vi "ADC Config Panel.vi"(8 "error in":errorcluster, 11 "adc session in":T2={"niScope"={"channel cfg"=[], "sessions"=[], "multi cards"=FALSE, "channels"=0, "type"=enum."n/a", "memory [B/chn]"=0, "ext. clock [Hz]"=0.0, "samples count"=0, "use streaming"=FALSE, "proc setup"={"packet size [smpl]"=0, "current timeout [s]"=0.0, "blk2blk timeout [s]"=0.0, "event time"=timestamp(0 s since 1904-01-01), "temp sampl T [s]"=0.0, "data queue"=refnum, "stop notifier"=refnum, "proc ref"=refnum}, "sample width [B]"=0, "ranges [V]"=[], "trigger setup"={"coupling"=1, "level [V]"=0.0, "slope"=0, "mode"=enum."Immediate"}, "fs [Hz]"=0.0, "bitres [bit]"=0}, "3458A"={"channels"=[], "sync unit"={"VISA"="", "type"=enum."Picotest U6200A"}, "awg unit"={"type"=enum."Agilent 331xxA to 332xxA", "VISA"="", "enable 10MHz ref"=FALSE}, "sync mode"=enum."MASTER-SLAVE, MASTER clocked by TIMER", "streaming mode"=FALSE, "idn mode"=enum."Auto", "sampling mode"=enum."DCV", "Ts [s]"=0.0, "sample memory [B]"=0, "proc setup"={"channel id"=0, "packet size [smpl]"=0, "current timeout [s]"=0.0, "blk2blk timeout [s]"=0.0, "event time"=timestamp(0 s since 1904-01-01), "stop notifier"=refnum, "data queues"=[], "proc refs"=[], "bus semaphore"=refnum}, "sample size [B]"=0, "sample count"=0, "aux data"={"channel id"=0, "valid?"=[], "gain [V]"=[], "timestamp [s]"=[], "Ts [s]"=0.0, "abs timestamp"=timestamp(0 s since 1904-01-01), "t [deg C]"=[]}, "ranges [V]"=[], "aperture [s]"=0.0, "LEVEL trigger"={"edge"=enum."POS", "level [V]"=0.0, "coupling"=enum."DC"}, "trigger mode"=enum."AUTO", "measure temp.?"=FALSE, "disp mesages"=[], "shared bus?"=FALSE, "disable display?"=FALSE, "aper mode"=enum."Manual", "aper rules"=[]}, "dsdll"={"dsdll"={"dsdll path"=path "", "dsdll handle"=[], "output devices"=[], "capture devices"=[]}, "channels"=0, "device id"=0, "channel idns"=[], "proc setup"={"packet size [smpl]"=0, "current timeout [s]"=0.0, "blk2blk timeout [s]"=0.0, "event time"=timestamp(0 s since 1904-01-01), "data queue"=refnum, "stop notifier"=refnum, "proc ref"=refnum}, "samples count"=0, "fs [Hz]"=0.0}, "type"=enum."niScope", "channel idn str"=[], "aux instr idn str"=[], "modified?"=FALSE, "simadc"={"channels"=[], "range [V]"=0.0, "Ts step [s]"=0.0, "time [s]"=0.0, "fs [Hz]"=0.0, "count"=0, "smpl offset"=0, "set count"=0, "bit res"=0}, "force rst?"=FALSE, "exit mode"=enum."Immediate reset", "exit dly"=0.0, "exit tmr"=timestamp(0 s since 1904-01-01), "busy?"=FALSE, "accessed?"=FALSE, "QuADC session"={"channel cfg"=[], "sessions"=[], "multi cards"=FALSE, "channels"=0, "type"=enum."n/a", "memory [B/chn]"=0, "ext. clock [Hz]"=0.0, "samples count"=0, "use streaming"=FALSE, "proc setup"={"packet size [smpl]"=0, "current timeout [s]"=0.0, "blk2blk timeout [s]"=0.0, "event time"=timestamp(0 s since 1904-01-01), "temp sampl T [s]"=0.0, "data queue"=refnum, "stop notifier"=refnum, "proc ref"=refnum}, "sample width [B]"=0, "ranges [V]"=[], "trigger setup"={"coupling"=1, "level [V]"=0.0, "slope"=0, "mode"=enum."Immediate"}, "fs [Hz]"=0.0, "bitres [bit]"=0}} {"QuADC session"."trigger setup"."level [V]" format="%.2f"; "QuADC session"."trigger setup"."coupling" items=["AC"=0, "DC"=1, "HF Reject"=3, "LF Reject"=4, "AC Plus HF Reject"=1001]; "QuADC session"."channel cfg"."Clock fr. (Hz)" min=0.0 format="%#_9p"; "QuADC session"."channel cfg"."Number of JJ" min=1; "QuADC session"."channel cfg"."Range [Vpk]" min=0.0; "QuADC session"."channel cfg"."Channel" min=0; "3458A"."channels"."Range [Vpk]" min=0.0; "niScope"."trigger setup"."level [V]" format="%.2f"; "niScope"."trigger setup"."coupling" items=["AC"=0, "DC"=1, "HF Reject"=3, "LF Reject"=4, "AC Plus HF Reject"=1001]; "niScope"."channel cfg"."Range [Vpk]" min=0.0; "niScope"."channel cfg"."Channel" min=0}) -> (0 "error out":errorcluster, 3 "adc session out":T2={"niScope"={"channel cfg"=[], "sessions"=[], "multi cards"=FALSE, "channels"=0, "type"=enum."n/a", "memory [B/chn]"=0, "ext. clock [Hz]"=0.0, "samples count"=0, "use streaming"=FALSE, "proc setup"={"packet size [smpl]"=0, "current timeout [s]"=0.0, "blk2blk timeout [s]"=0.0, "event time"=timestamp(0 s since 1904-01-01), "temp sampl T [s]"=0.0, "data queue"=refnum, "stop notifier"=refnum, "proc ref"=refnum}, "sample width [B]"=0, "ranges [V]"=[], "trigger setup"={"coupling"=1, "level [V]"=0.0, "slope"=0, "mode"=enum."Immediate"}, "fs [Hz]"=0.0, "bitres [bit]"=0}, "3458A"={"channels"=[], "sync unit"={"VISA"="", "type"=enum."Picotest U6200A"}, "awg unit"={"type"=enum."Agilent 331xxA to 332xxA", "VISA"="", "enable 10MHz ref"=FALSE}, "sync mode"=enum."MASTER-SLAVE, MASTER clocked by TIMER", "streaming mode"=FALSE, "idn mode"=enum."Auto", "sampling mode"=enum."DCV", "Ts [s]"=0.0, "sample memory [B]"=0, "proc setup"={"channel id"=0, "packet size [smpl]"=0, "current timeout [s]"=0.0, "blk2blk timeout [s]"=0.0, "event time"=timestamp(0 s since 1904-01-01), "stop notifier"=refnum, "data queues"=[], "proc refs"=[], "bus semaphore"=refnum}, "sample size [B]"=0, "sample count"=0, "aux data"={"channel id"=0, "valid?"=[], "gain [V]"=[], "timestamp [s]"=[], "Ts [s]"=0.0, "abs timestamp"=timestamp(0 s since 1904-01-01), "t [deg C]"=[]}, "ranges [V]"=[], "aperture [s]"=0.0, "LEVEL trigger"={"edge"=enum."POS", "level [V]"=0.0, "coupling"=enum."DC"}, "trigger mode"=enum."AUTO", "measure temp.?"=FALSE, "disp mesages"=[], "shared bus?"=FALSE, "disable display?"=FALSE, "aper mode"=enum."Manual", "aper rules"=[]}, "dsdll"={"dsdll"={"dsdll path"=path "", "dsdll handle"=[], "output devices"=[], "capture devices"=[]}, "channels"=0, "device id"=0, "channel idns"=[], "proc setup"={"packet size [smpl]"=0, "current timeout [s]"=0.0, "blk2blk timeout [s]"=0.0, "event time"=timestamp(0 s since 1904-01-01), "data queue"=refnum, "stop notifier"=refnum, "proc ref"=refnum}, "samples count"=0, "fs [Hz]"=0.0}, "type"=enum."niScope", "channel idn str"=[], "aux instr idn str"=[], "modified?"=FALSE, "simadc"={"channels"=[], "range [V]"=0.0, "Ts step [s]"=0.0, "time [s]"=0.0, "fs [Hz]"=0.0, "count"=0, "smpl offset"=0, "set count"=0, "bit res"=0}, "force rst?"=FALSE, "exit mode"=enum."Immediate reset", "exit dly"=0.0, "exit tmr"=timestamp(0 s since 1904-01-01), "busy?"=FALSE, "accessed?"=FALSE, "QuADC session"={"channel cfg"=[], "sessions"=[], "multi cards"=FALSE, "channels"=0, "type"=enum."n/a", "memory [B/chn]"=0, "ext. clock [Hz]"=0.0, "samples count"=0, "use streaming"=FALSE, "proc setup"={"packet size [smpl]"=0, "current timeout [s]"=0.0, "blk2blk timeout [s]"=0.0, "event time"=timestamp(0 s since 1904-01-01), "temp sampl T [s]"=0.0, "data queue"=refnum, "stop notifier"=refnum, "proc ref"=refnum}, "sample width [B]"=0, "ranges [V]"=[], "trigger setup"={"coupling"=1, "level [V]"=0.0, "slope"=0, "mode"=enum."Immediate"}, "fs [Hz]"=0.0, "bitres [bit]"=0}} {"QuADC session"."trigger setup"."level [V]" format="%.2f"; "QuADC session"."trigger setup"."coupling" items=["AC"=0, "DC"=1, "HF Reject"=3, "LF Reject"=4, "AC Plus HF Reject"=1001]; "QuADC session"."channel cfg"."Clock fr. (Hz)" min=0.0 format="%#_9p"; "QuADC session"."channel cfg"."Number of JJ" min=1; "QuADC session"."channel cfg"."Range [Vpk]" min=0.0; "QuADC session"."channel cfg"."Channel" min=0; "3458A"."channels"."Range [Vpk]" min=0.0; "niScope"."trigger setup"."level [V]" format="%.2f"; "niScope"."trigger setup"."coupling" items=["AC"=0, "DC"=1, "HF Reject"=3, "LF Reject"=4, "AC Plus HF Reject"=1001]; "niScope"."channel cfg"."Range [Vpk]" min=0.0; "niScope"."channel cfg"."Channel" min=0})   [LabVIEW 2018]
doc: "Configuration panel for digitizer."
uses:
  drivers/niScope/niScope Virtual Channel Config.ctl
  drivers/niScope/niScope Virtual Channel Mode.ctl
  drivers/niScope/niScope Virtual Channel Input Z.ctl
  drivers/niScope/niScope Virtual Channel Coupling.ctl
  ADC Type.ctl
  drivers/DMM/3458A Virtual Channel Config.ctl
  drivers/AWG/AWG Type.ctl
  drivers/DMM/3458A Idn Mode.ctl
  drivers/Counter/Counter Type.ctl
  drivers/DMM/3458A Digitizing Low Levels/Configure/Sampling Mode.ctl
  drivers/DMM/3458A Sync Mode.ctl
  ADC Session.ctl
  drivers/niScope/niScope Session.ctl
  drivers/niScope/niScope Type.ctl
  drivers/niScope/niScope Digitizing Process Options.ctl
  drivers/niScope/niScope Data Packet.ctl
  drivers/niScope/niScope Trigger Setup.ctl
  <instrlib>/niScope/Controls/niScope trigger coupling.ctl
  <instrlib>/niScope/Controls/niScope trigger slope.ctl
  drivers/DMM/3458A Digitizer Session.ctl
  drivers/Counter/Counter Session.ctl
  drivers/AWG/AWG Session.ctl
  drivers/DMM/3458A Digitizing Process Options.ctl
  drivers/DMM/3458A Data Packet.ctl
  drivers/DMM/3458A Aux Record Data.ctl
  drivers/DMM/3458A Digitizing Low Levels/Configure/Level Setup.ctl
  drivers/DMM/3458A Digitizing Low Levels/Configure/First Sample Trigger.ctl
  drivers/DMM/3458A Aperture Selection Mode.ctl
  drivers/dsdll/DSDLL Session.ctl
  drivers/dsdll/dsdll source distribution/dsdll_instance.ctl
  drivers/dsdll/dsdll source distribution/dsdll_device_record.ctl
  drivers/dsdll/DSDLL Process Config.ctl
  drivers/dsdll/DSDLL Data Packet.ctl
  drivers/simulated_adc/SimAdc Config.ctl
  drivers/simulated_adc/SimAdc Channel Cfg.ctl
  ADC On Close Action.ctl
  drivers/Quatsch_driver/QuADCDriver/QuADC Session.ctl
  drivers/Quatsch_driver/QuADCDriver/QuADC Virtual Channel Config.ctl
  drivers/Quatsch_driver/QuADCDriver/QuADC Virtual Channel Mode.ctl
  drivers/Quatsch_driver/QuADCDriver/QuADC Virtual Channel Input Z.ctl
  drivers/Quatsch_driver/QuADCDriver/QuADC Virtual Channel Coupling.ctl
  drivers/Quatsch_driver/QuADCDriver/QuADC Type.ctl
  drivers/Quatsch_driver/QuADCDriver/QuADC Digitizing Process Options.ctl
  drivers/Quatsch_driver/QuADCDriver/QuADC Data Packet.ctl
  drivers/Quatsch_driver/QuADCDriver/QuADC Trigger Setup.ctl
  varilib/SGUI Assign References Mode.ctl
  varilib/SGUI Assign Multiple Strings With Tags By Label.vi
  drivers/DMM/3458A Virtual Digitizer.lvlib
  drivers/Counter/Counter.lvlib
  drivers/AWG/AWG.lvlib
  drivers/DMM/3458A Digitizing Low Levels/3458A Digitizing Low Levels.lvlib
  varilib/varilib.lvlib
  drivers/niScope/niScope Virtual Digitizer.lvlib
  drivers/dsdll/DSDLL Virtual Digitizer.lvlib
  drivers/Quatsch_driver/QuADCDriver/QuADC Virtual Digitizer.lvlib
  drivers/dsdll/dsdll source distribution/dsdll.lvlib
panel:
  in  "tc on exit":enum32{"Page 1"}(tab)
  in  "exit delay":dbl=30.0 caption="Delay [s]"
  in  "exit mode":T1 caption="On device close"
  in  "force rst":bool caption="Force reset on open"
  in  "btn selfcal":bool
  in  "tc idn":enum32{"Page 1"}(tab)
  out "adcstr":string caption="Identification/Status:"
  in  "btn test":bool
  in  "btn cancel":bool
  in  "btn ok":bool
  in  "tc type":enum32{"Page 1"}(tab)
  out "Description":string
  in  "Digitizer type":T32
  in  "tc cfg":T43(tab)
  in  "btn rem last niScope":bool
  in  "niSc streaming":bool caption="Use streaming mode"
  in  "niSc ext clock":dbl caption="External clock [Hz]" format="%#_6p"
  in  "btn clr niScope":bool
  in  "niSc channels":T4[](array[typedef]) caption="ADC Channels" {"Range [Vpk]" min=0.0; "Channel" min=0}
  in  "dmm aper mode":T27 caption="Aperture selection mode"
  in  "dmm aper rules":string[][](table) caption="Aperture auto selection rules"
  in  "dmm disable disp":bool caption="Disable display"
  in  "btn rem last dmm":bool
  in  "dmm meas t":bool caption="Measure temperature"
  in  "dmm stream":bool caption="Use streaming mode"
  in  "dmm sync mode":T19 caption="Synchronization mode"
  in  "counter VISA":refnum<visa-resource-name> caption="Counter VISA"
  in  "AWG VISA":refnum<visa-resource-name>
  in  "counter type":T16 caption="Counter type"
  in  "AWG ext ref":bool caption="Use external 10 MHz for AWG"
  in  "AWG type":T18
  in  "DMM Channels":T14[](array[typedef]) {"Range [Vpk]" min=0.0}
  in  "btn clr dmm":bool
  in  "dmm idn mode":T20 caption="DMM descriptor mode"
  in  "dmm smpl mode":T21 caption="DMM digitizing mode"
  in  "btn dsdll enum":bool
  in  "dsdll channels":i32=1 caption="Channels count (1 or 2)" min=1 max=2 step=1
  in  "dsdll capt devs":u16(ring) caption="Capture devices"
  in  "simadc bitres":i32=16 caption="ADC resolution [bit]"
  in  "Range [V]":dbl
  in  "Sampling period step [s]":dbl
  in  "btn sim clr":bool caption="Clear List"
  in  "simadc chn cfg":T34[](array[typedef]) caption="Channel signal definitions"
  in  "QuADC channels":T36[](array[typedef])=[{"Channel"=0, "Mode"=enum."Single ended", "Input Z"=enum."1 MOhm", "Coupling"=enum."DC", "Range [Vpk]"=1.0, "btn clr"=FALSE, "btn up"=FALSE, "btn down"=FALSE, "IP address A"=127, "IP address B"=0, "IP address C"=0, "IP address D"=1, "Port"=8888, "Number of JJ"=1000, "Clock fr. (Hz)"=5000000000.0}] {"Clock fr. (Hz)" min=0.0 format="%#_9p"; "Number of JJ" min=1; "Range [Vpk]" min=0.0; "Channel" min=0}
  # "IP Address"
  # "."
  # "."
  # "."
  # ":"
  # "IP Address"
  # "."
  # "."
  # "."
  # ":"
  # "- Use 0 for internal clock"
  # "Streaming mode is used always."
  # "IP Address"
  # "."
  # "."
  # "."
  # ":"
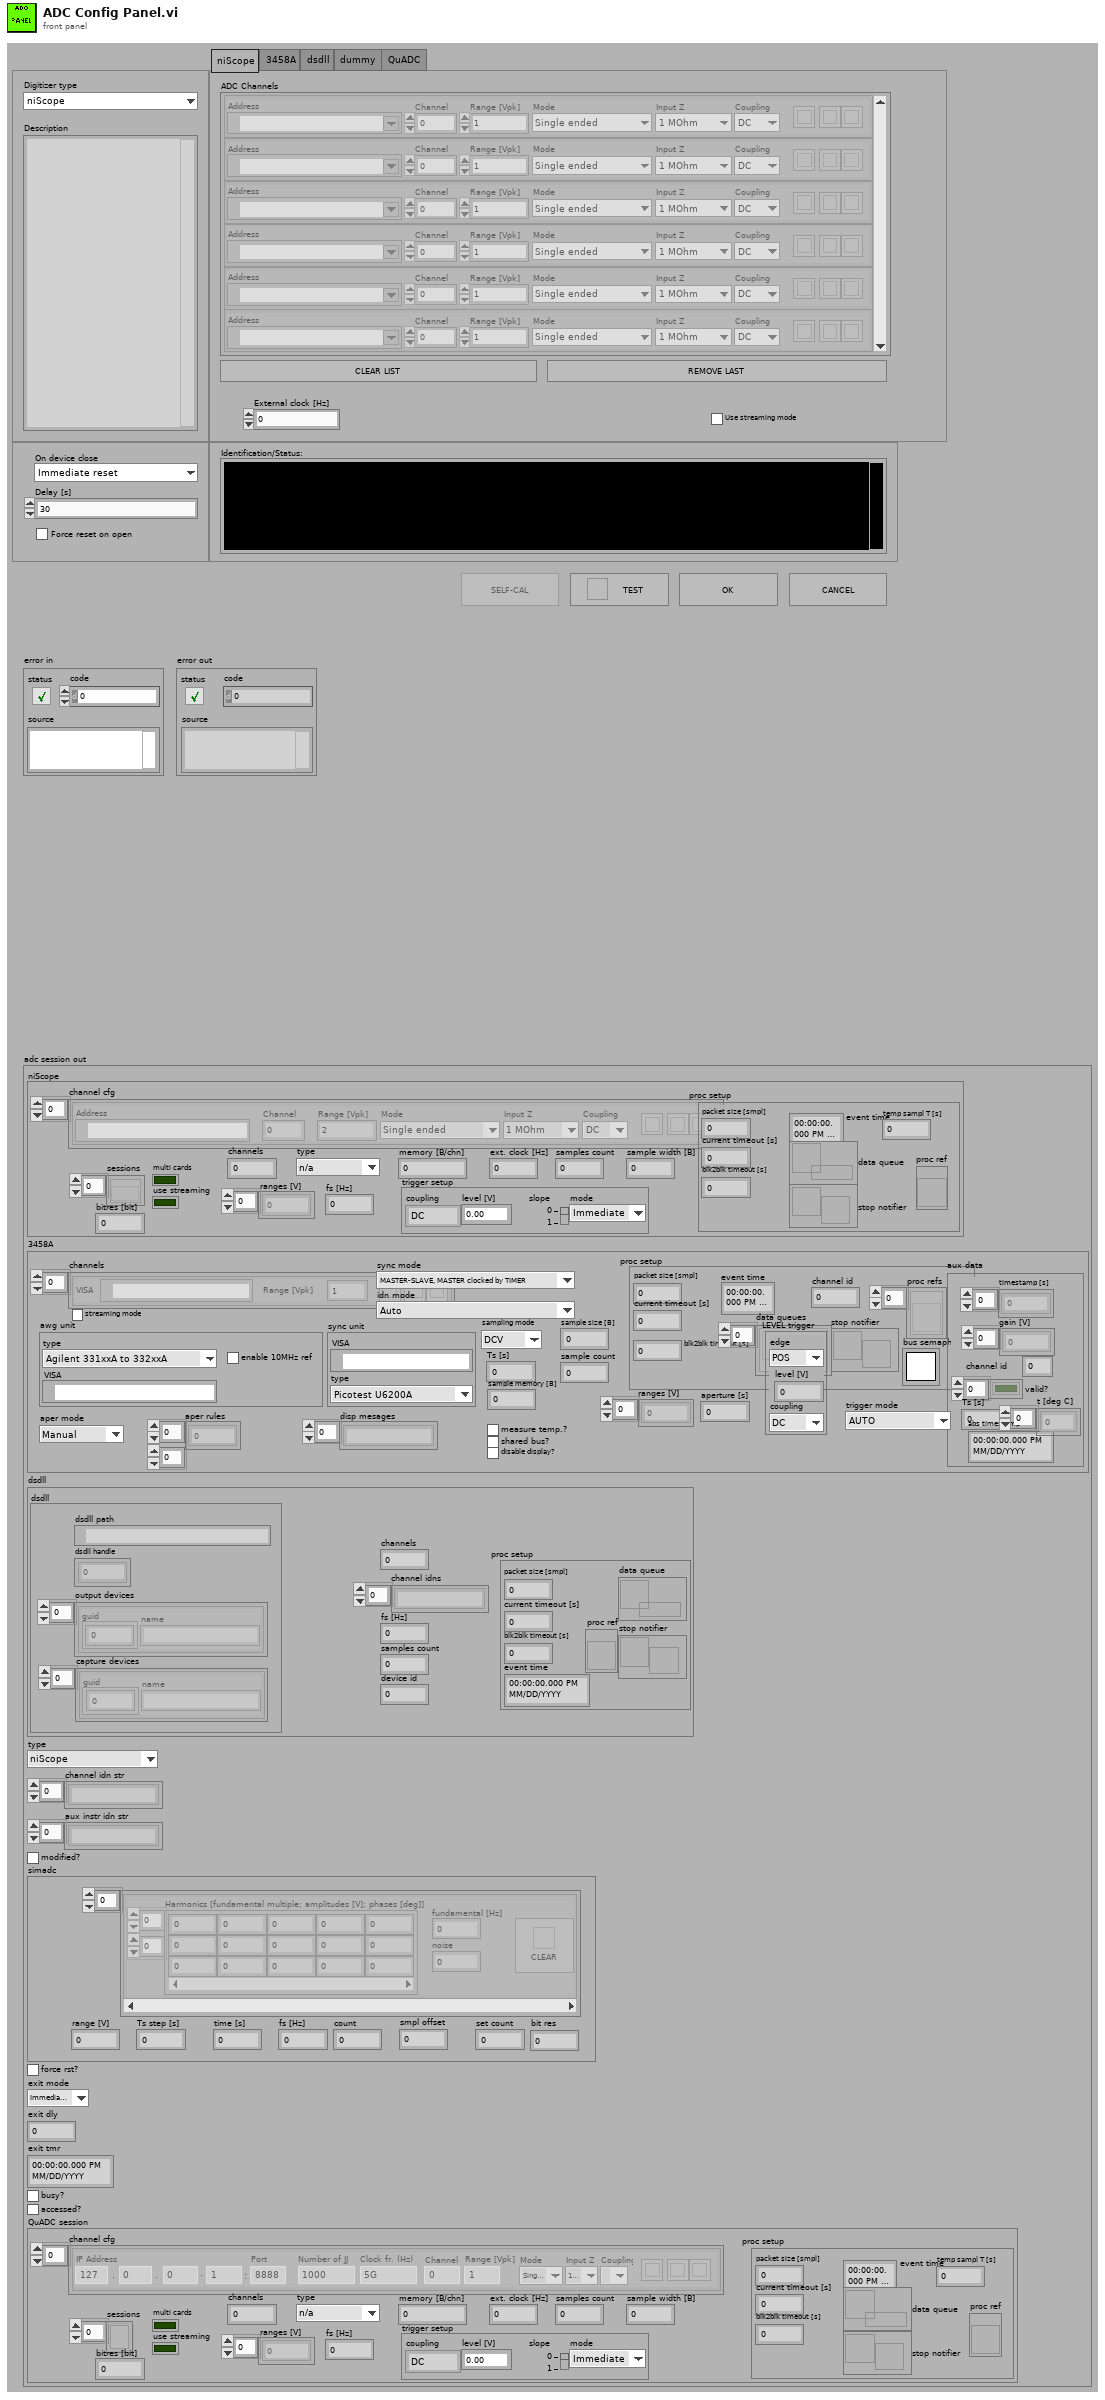
[diagram p1: front panel]
types:
  T1 = typedef "ADC On Close Action.ctl" = enum16{"Immediate reset", "Delayed reset"}
  T2 = typedef "ADC Session.ctl" = cluster{"niScope":T3, "3458A":T13, "dsdll":T28, "type":T32, "channel idn str":string[], "aux instr idn str":string[], "modified?":bool, "simadc":T33, "force rst?":bool, "exit mode":T1, "exit dly":dbl, "exit tmr":timestamp, "busy?":bool, "accessed?":bool, "QuADC session":T35}
  T3 = typedef "niScope Virtual Digitizer.lvlib/niScope Session.ctl" = cluster{"channel cfg":T4[], "sessions":refnum<k20>[], "multi cards":bool, "channels":i32, "type":T8, "memory [B/chn]":i32, "ext. clock [Hz]":dbl, "samples count":i64, "use streaming":bool, "proc setup":T9, "sample width [B]":i32, "ranges [V]":dbl[], "trigger setup":T10, "fs [Hz]":dbl, "bitres [bit]":i32}
  T4 = typedef "niScope Virtual Digitizer.lvlib/niScope Virtual Channel Config.ctl" = cluster{"Address":refnum<k15>, "Channel":i32, "Mode":T5, "Input Z":T6, "Coupling":T7, "Range [Vpk]":dbl, "btn clr":bool, "btn up":bool, "btn down":bool}
  T5 = typedef "niScope Virtual Digitizer.lvlib/niScope Virtual Channel Mode.ctl" = enum16{"Single ended", "Unbal. differential", "Differential"}
  T6 = typedef "niScope Virtual Digitizer.lvlib/niScope Virtual Channel Input Z.ctl" = enum16{"1 MOhm", "50 Ohm"}
  T7 = typedef "niScope Virtual Digitizer.lvlib/niScope Virtual Channel Coupling.ctl" = enum16{"AC", "DC", "GND"}
  T8 = typedef "niScope Virtual Digitizer.lvlib/niScope Type.ctl" = enum16{"n/a", "5922"}
  T9 = typedef "niScope Virtual Digitizer.lvlib/niScope Digitizing Process Options.ctl" = cluster{"packet size [smpl]":i64, "current timeout [s]":dbl, "blk2blk timeout [s]":dbl, "event time":timestamp, "temp sampl T [s]":dbl, "data queue":refnum<queue>, "stop notifier":refnum<notifier>, "proc ref":refnum<vi>}
  T10 = typedef "niScope Virtual Digitizer.lvlib/niScope Trigger Setup.ctl" = cluster{"coupling":T11, "level [V]":dbl, "slope":T12, "mode":enum16{"Immediate", "External", "Level"}}
  T11 = typedef "niScope trigger coupling.ctl" = u16
  T12 = typedef "niScope trigger slope.ctl" = i32
  T13 = typedef "3458A Virtual Digitizer.lvlib/3458A Digitizer Session.ctl" = cluster{"channels":T14[], "sync unit":T15, "awg unit":T17, "sync mode":T19, "streaming mode":bool, "idn mode":T20, "sampling mode":T21, "Ts [s]":dbl, "sample memory [B]":i32, "proc setup":T22, "sample size [B]":i32, "sample count":i32, "aux data":T24, "ranges [V]":dbl[], "aperture [s]":dbl, "LEVEL trigger":T25, "trigger mode":T26, "measure temp.?":bool, "disp mesages":string[], "shared bus?":bool, "disable display?":bool, "aper mode":T27, "aper rules":dbl[][]}
  T14 = typedef "3458A Virtual Digitizer.lvlib/3458A Virtual Channel Config.ctl" = cluster{"VISA":refnum<visa-resource-name>, "Range [Vpk]":dbl, "btn clr":bool, "btn up":bool, "btn down":bool}
  T15 = typedef "Counter.lvlib/Counter Session.ctl" = cluster{"VISA":refnum<visa-resource-name>, "type":T16}
  T16 = typedef "Counter.lvlib/Counter Type.ctl" = enum16{"Picotest U6200A", "dummy"}
  T17 = typedef "AWG.lvlib/AWG Session.ctl" = cluster{"type":T18, "VISA":refnum<visa-resource-name>, "enable 10MHz ref":bool}
  T18 = typedef "AWG.lvlib/AWG Type.ctl" = enum16{"Agilent 331xxA to 332xxA", "Agilent 335xxA to 336xxA", "Tektronix AFG3101C", "dummy"}
  T19 = typedef "3458A Virtual Digitizer.lvlib/3458A Sync Mode.ctl" = enum16{"MASTER-SLAVE, MASTER clocked by TIMER", "MASTER-SLAVE, MASTER clocked by AWG", "ALL clocked by AWG", "MASTER-SLAVE, ALL clocked by TIMER", "ALL clocked by AWG with DFLL"}
  T20 = typedef "3458A Virtual Digitizer.lvlib/3458A Idn Mode.ctl" = enum16{"Auto", "Sequential (chn A, chn B, ...)", "From calibration string"}
  T21 = typedef "3458A Virtual Digitizer.lvlib/3458A Digitizing Low Levels.lvlib/Sampling Mode.ctl" = enum16{"DCV", "DSDC", "DSAC"}
  T22 = typedef "3458A Virtual Digitizer.lvlib/3458A Digitizing Process Options.ctl" = cluster{"channel id":i32, "packet size [smpl]":i32, "current timeout [s]":dbl, "blk2blk timeout [s]":dbl, "event time":timestamp, "stop notifier":refnum<notifier>, "data queues":refnum<queue>[], "proc refs":refnum<vi>[], "bus semaphore":T23}
  T23 = typedef "Semaphore RefNum" = refnum<k1>
  T24 = typedef "3458A Virtual Digitizer.lvlib/3458A Aux Record Data.ctl" = cluster{"channel id":i32, "valid?":bool[], "gain [V]":dbl[], "timestamp [s]":dbl[], "Ts [s]":dbl, "abs timestamp":timestamp, "t [deg C]":dbl[]}
  T25 = typedef "3458A Virtual Digitizer.lvlib/3458A Digitizing Low Levels.lvlib/Level Setup.ctl" = cluster{"edge":enum16{"POS", "NEG"}, "level [V]":dbl, "coupling":enum16{"DC", "AC"}}
  T26 = typedef "3458A Virtual Digitizer.lvlib/3458A Digitizing Low Levels.lvlib/First Sample Trigger.ctl" = enum16{"AUTO", "EXT", "SYN", "SGL", "HOLD", "LEVEL"}
  T27 = typedef "3458A Virtual Digitizer.lvlib/3458A Aperture Selection Mode.ctl" = enum16{"Manual", "Maximum", "Table"}
  T28 = typedef "DSDLL Virtual Digitizer.lvlib/DSDLL Session.ctl" = cluster{"dsdll":T29, "channels":i32, "device id":i32, "channel idns":string[], "proc setup":T31, "samples count":i32, "fs [Hz]":dbl}
  T29 = typedef "dsdll.lvlib/dsdll_instance.ctl" = cluster{"dsdll path":path, "dsdll handle":u8[], "output devices":T30[], "capture devices":T30[]}
  T30 = typedef "dsdll.lvlib/dsdll_device_record.ctl" = cluster{"guid":u8[], "name":string}
  T31 = typedef "DSDLL Virtual Digitizer.lvlib/DSDLL Process Config.ctl" = cluster{"packet size [smpl]":i32, "current timeout [s]":dbl, "blk2blk timeout [s]":dbl, "event time":timestamp, "data queue":refnum<queue>, "stop notifier":refnum<notifier>, "proc ref":refnum<vi>}
  T32 = typedef "ADC Type.ctl" = enum16{"niScope", "3458A", "DirectSound DLL", "dummy", "QuADC"}
  T33 = typedef "SimAdc Config.ctl" = cluster{"channels":T34[], "range [V]":dbl, "Ts step [s]":dbl, "time [s]":dbl, "fs [Hz]":dbl, "count":i64, "smpl offset":i64, "set count":i64, "bit res":i32}
  T34 = typedef "SimAdc Channel Cfg.ctl" = cluster{"harmonics":dbl[][], "btn clear":bool, "noise":dbl, "fundamental [Hz]":dbl}
  T35 = typedef "QuADC Virtual Digitizer.lvlib/QuADC Session.ctl" = cluster{"channel cfg":T36[], "sessions":refnum<k5>[], "multi cards":bool, "channels":i32, "type":T40, "memory [B/chn]":i32, "ext. clock [Hz]":dbl, "samples count":i64, "use streaming":bool, "proc setup":T41, "sample width [B]":i32, "ranges [V]":dbl[], "trigger setup":T42, "fs [Hz]":dbl, "bitres [bit]":i32}
  T36 = typedef "QuADC Virtual Digitizer.lvlib/QuADC Virtual Channel Config.ctl" = cluster{"Channel":i32, "Mode":T37, "Input Z":T38, "Coupling":T39, "Range [Vpk]":dbl, "btn clr":bool, "btn up":bool, "btn down":bool, "IP address A":u8, "IP address B":u8, "IP address C":u8, "IP address D":u8, "Port":u16, "Number of JJ":u32, "Clock fr. (Hz)":dbl}
  T37 = typedef "QuADC Virtual Digitizer.lvlib/QuADC Virtual Channel Mode.ctl" = enum16{"Single ended", "Unbal. differential", "Differential"}
  T38 = typedef "QuADC Virtual Digitizer.lvlib/QuADC Virtual Channel Input Z.ctl" = enum16{"1 MOhm", "50 Ohm"}
  T39 = typedef "QuADC Virtual Digitizer.lvlib/QuADC Virtual Channel Coupling.ctl" = enum16{"AC", "DC", "GND"}
  T40 = typedef "QuADC Virtual Digitizer.lvlib/QuADC Type.ctl" = enum16{"n/a", "v1"}
  T41 = typedef "QuADC Virtual Digitizer.lvlib/QuADC Digitizing Process Options.ctl" = cluster{"packet size [smpl]":i64, "current timeout [s]":dbl, "blk2blk timeout [s]":dbl, "event time":timestamp, "temp sampl T [s]":dbl, "data queue":refnum<queue>, "stop notifier":refnum<notifier>, "proc ref":refnum<vi>}
  T42 = typedef "QuADC Virtual Digitizer.lvlib/QuADC Trigger Setup.ctl" = cluster{"coupling":T11, "level [V]":dbl, "slope":T12, "mode":enum16{"Immediate", "External", "Level"}}
  T43 = enum32{"niScope", "3458A", "dsdll", "dummy", "QuADC"}
  T44 = typedef "varilib.lvlib/SGUI Assign References Mode.ctl" = enum16{"Add to stack", "Overwrite", "Release last", "Release ID"}
  T45 = typedef "ADC Capabilities.ctl" = cluster{"max samples count":i64, "max fs [Hz]":ext, "min fs [Hz]":ext, "Ts step [s]":ext, "max Ts [s]":ext, "min Ts [s]":ext, "allows streaming?":bool, "streaming on?":bool, "has level trig?":bool, "has ext trig?":bool, "has aperture?":bool, "aper min [s]":dbl, "aper max [s]":dbl, "channels count":i32, "has ranges?":bool, "has temperature?":bool, "has temperature log?":bool, "has selfcal?":bool, "fs step [Hz]":ext, "smpl rate step mode":T46}
  T46 = typedef "ADC Sampling Rate Step Mode.ctl" = enum16{"const period", "const frequency"}
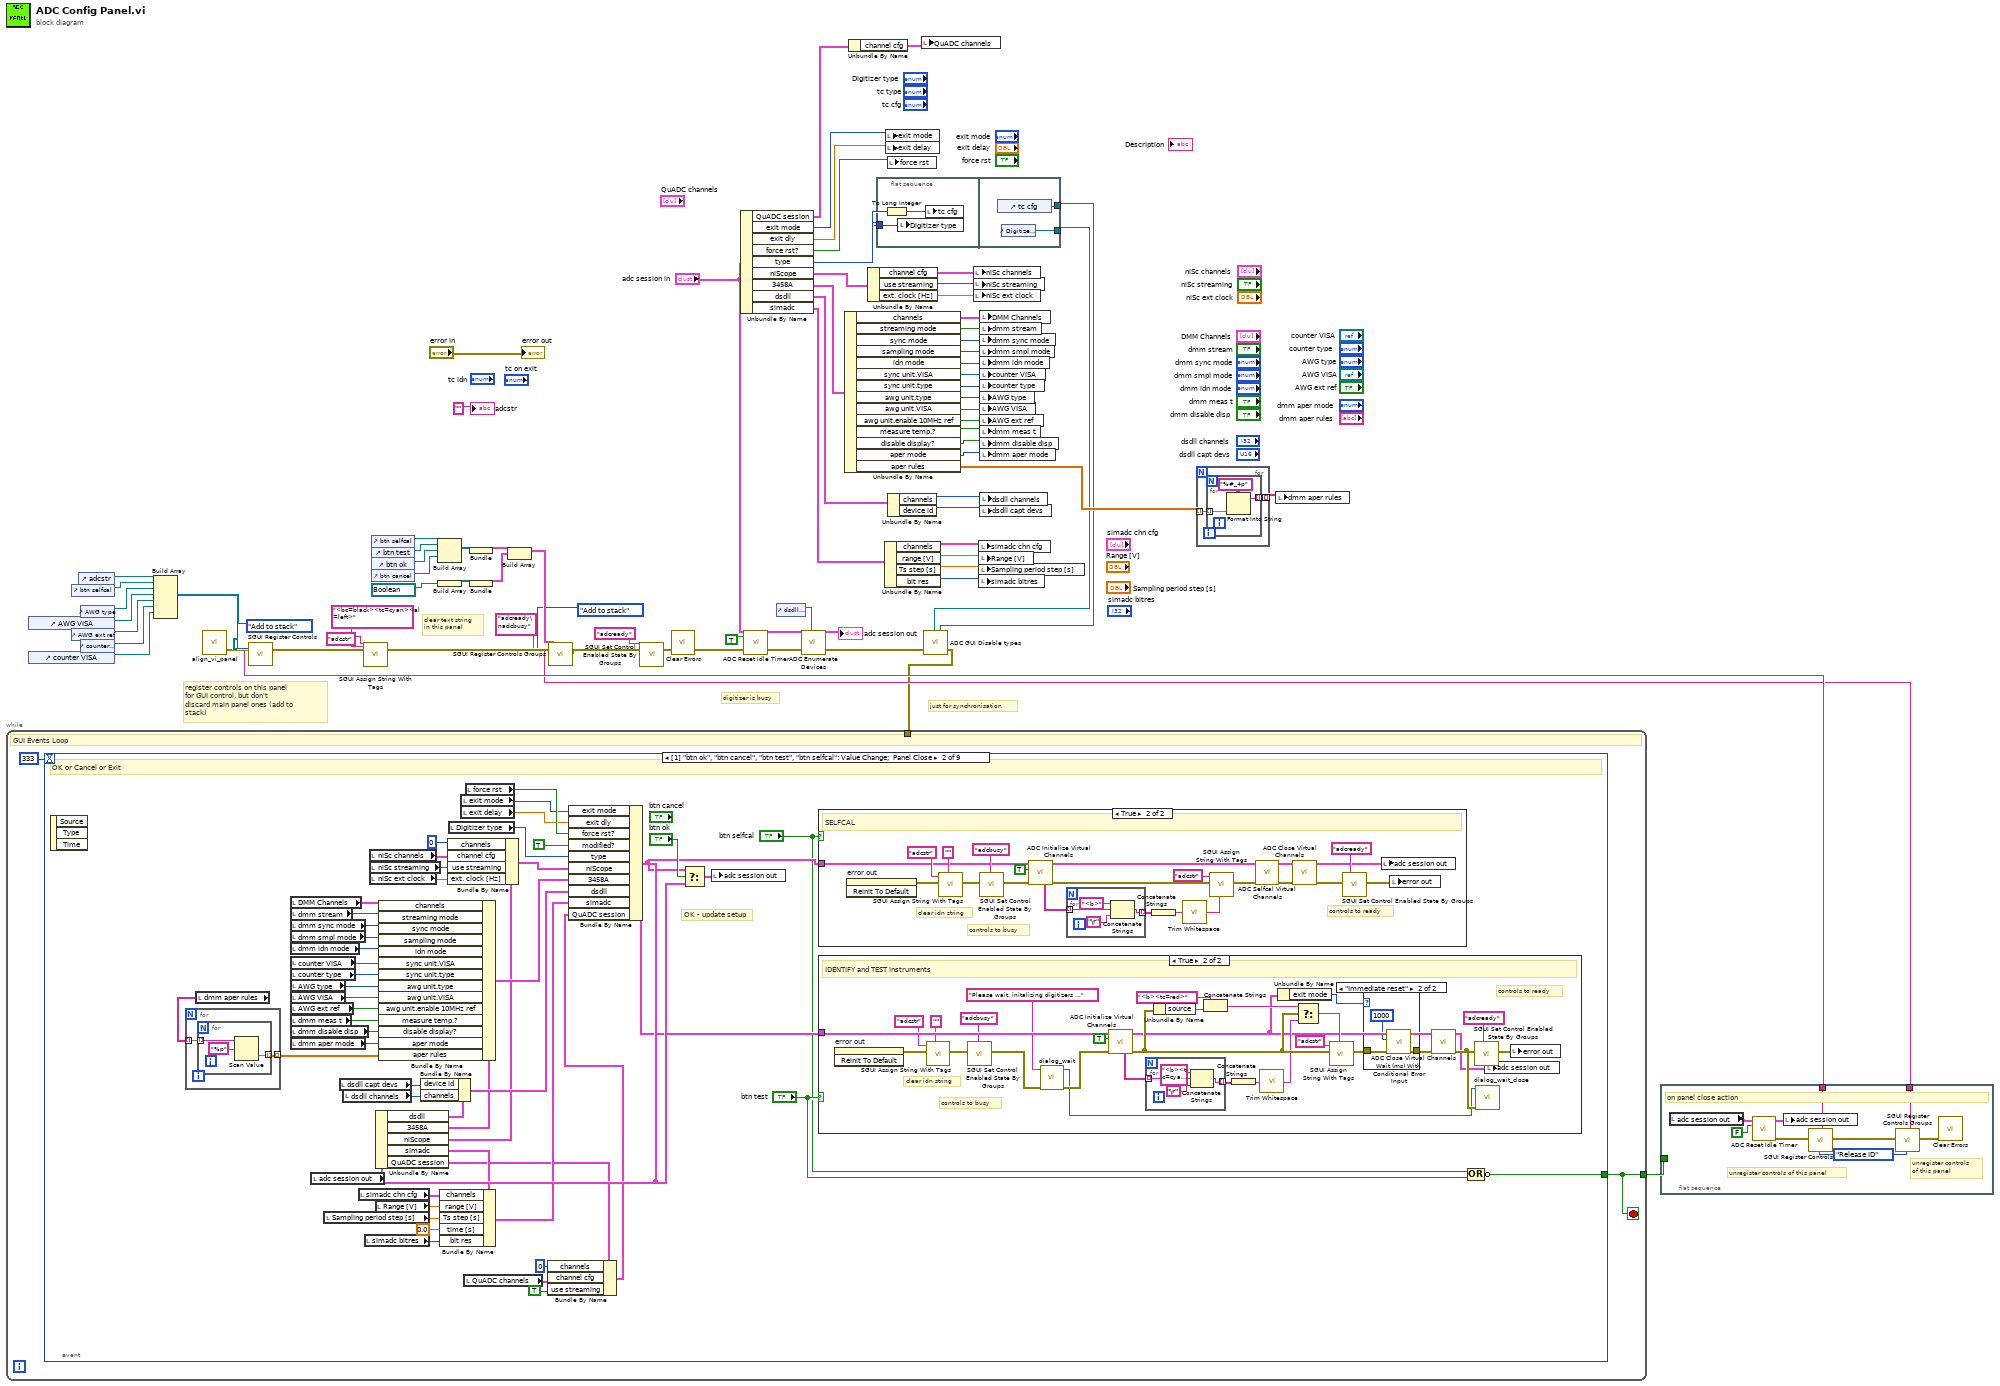
[diagram p0: block diagram]
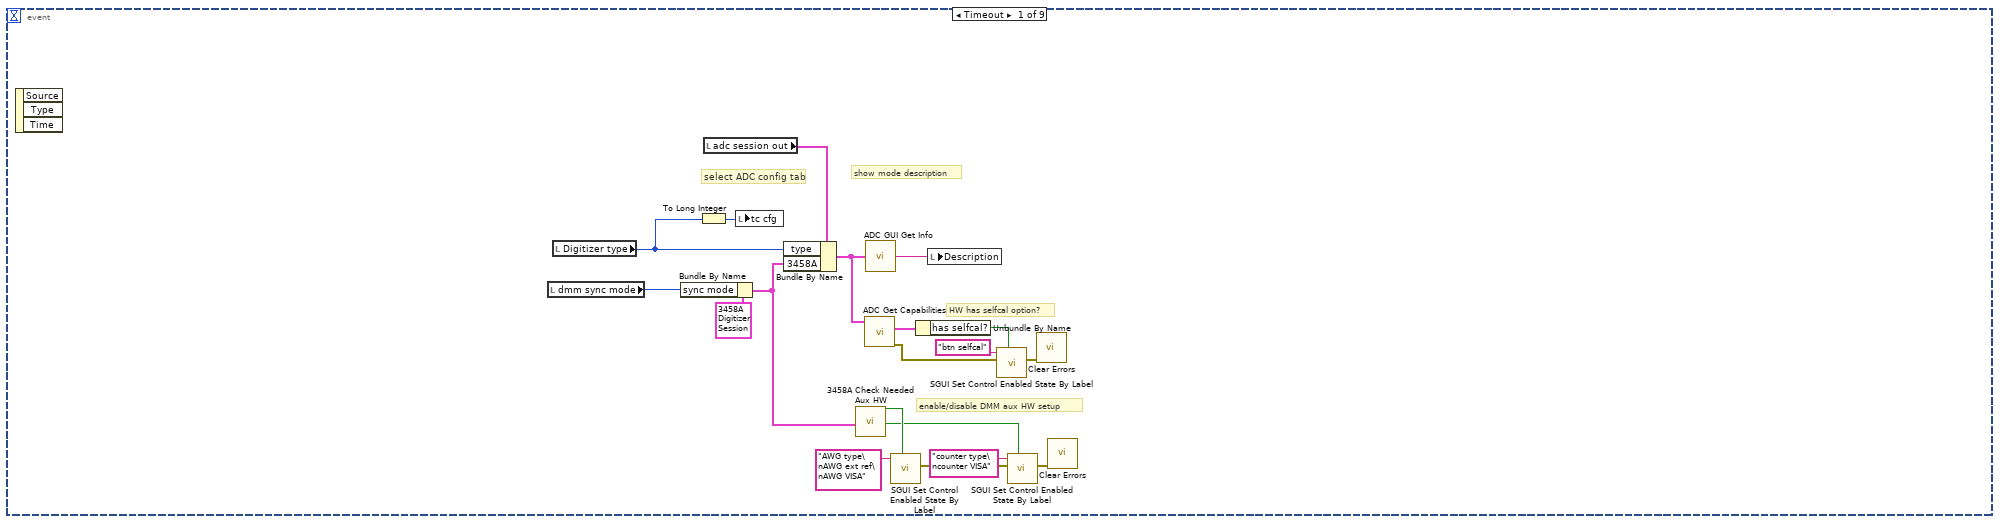
[diagram p2: hidden frame]
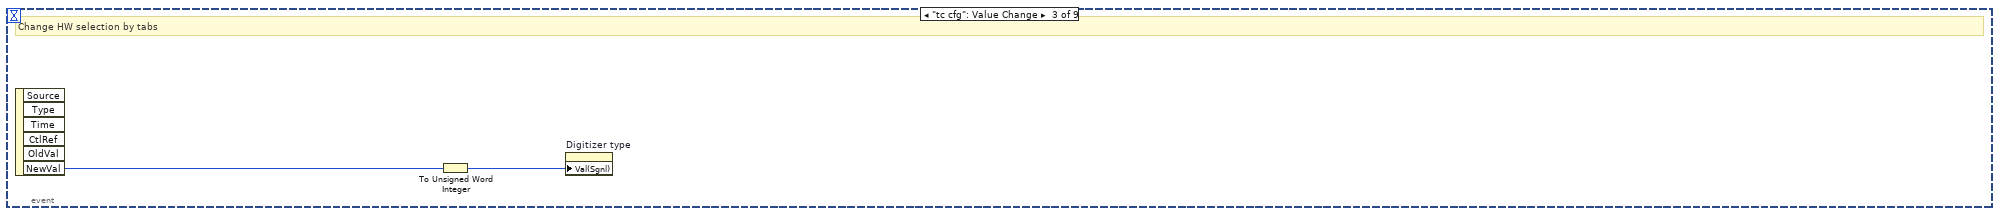
[diagram p6: hidden frame]
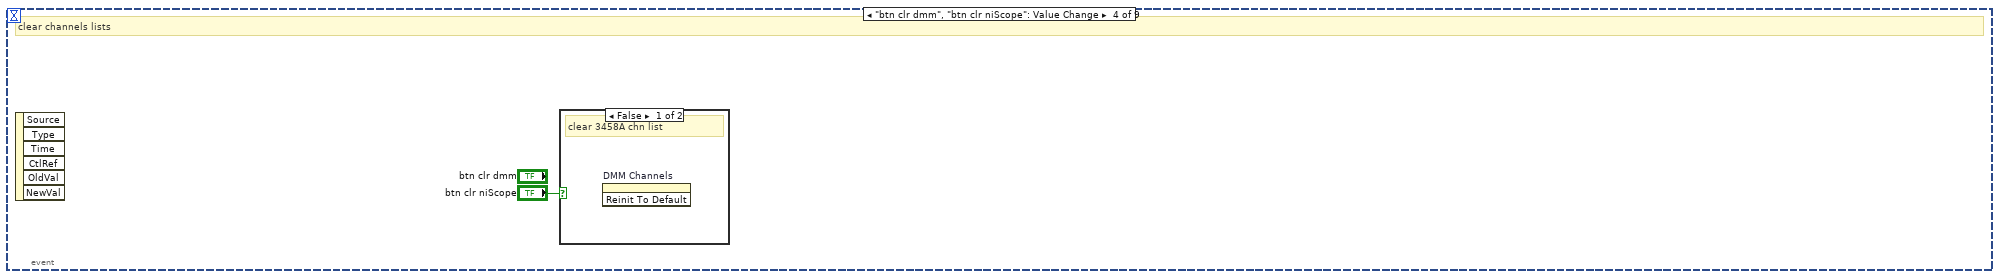
[diagram p7: hidden frame]
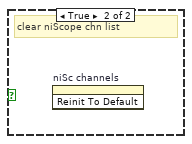
[diagram p8: hidden frame]
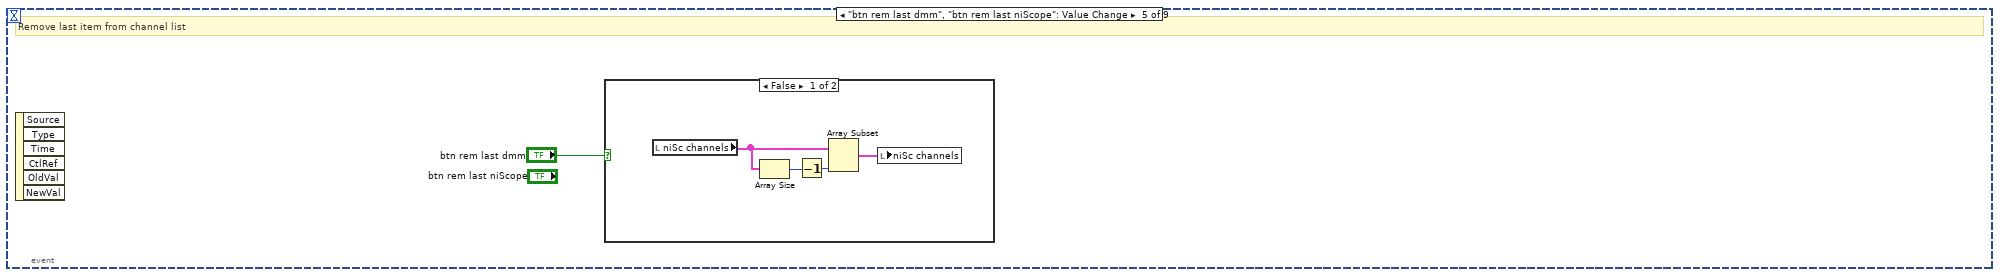
[diagram p9: hidden frame]
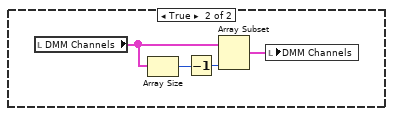
[diagram p10: hidden frame]
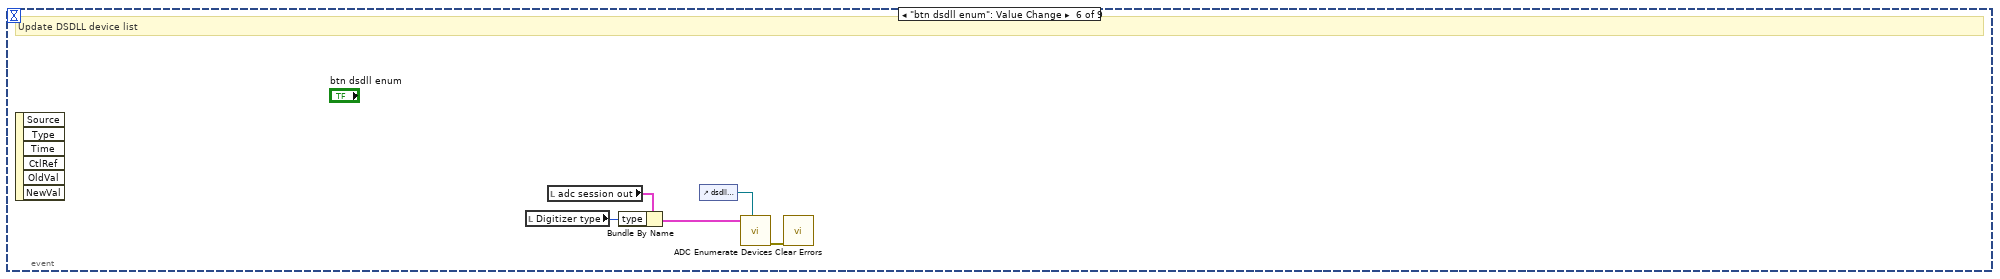
[diagram p11: hidden frame]
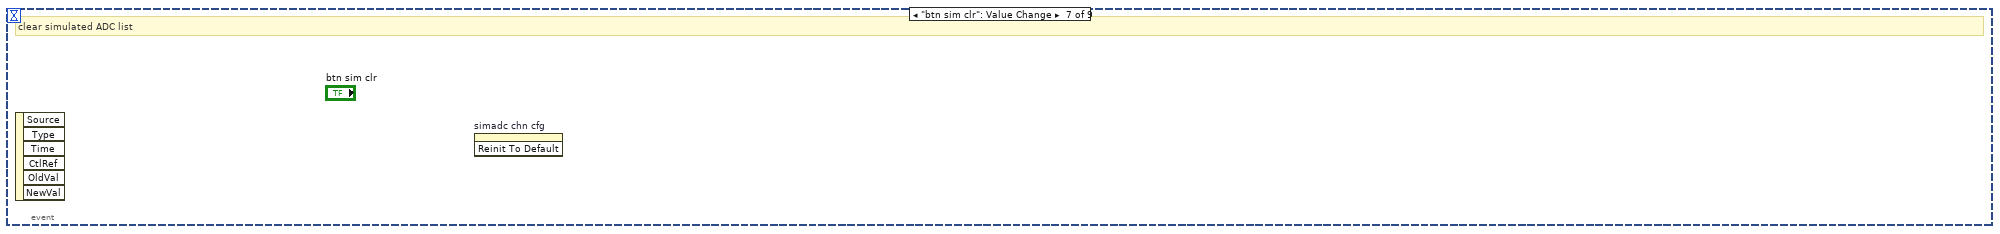
[diagram p12: hidden frame]
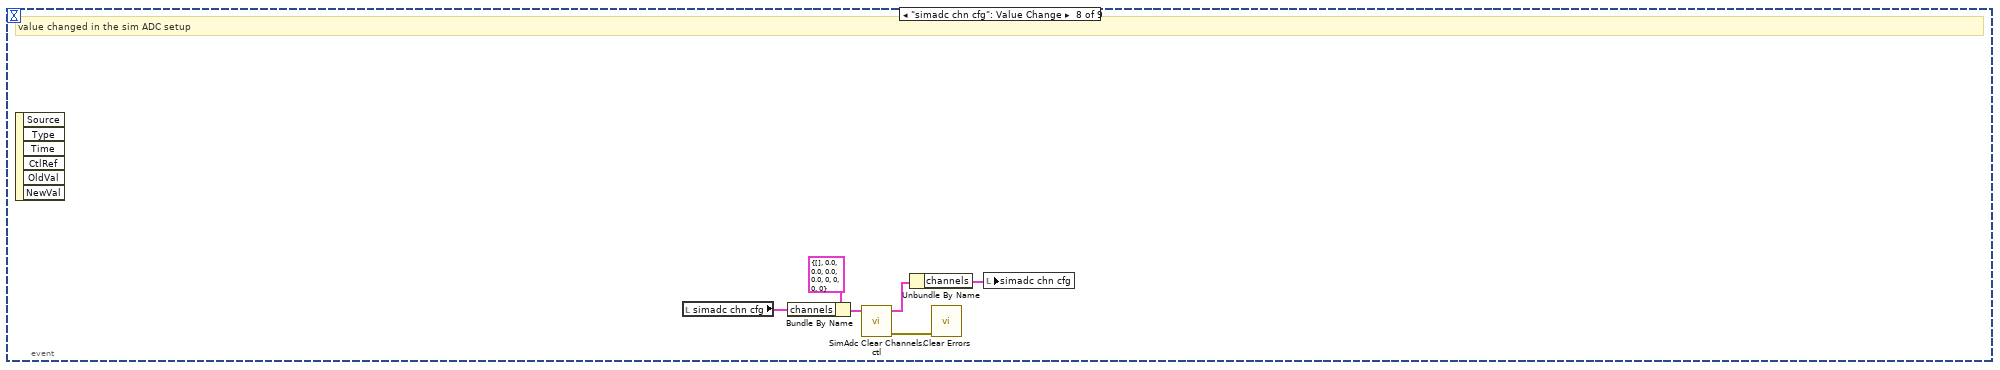
[diagram p13: hidden frame]
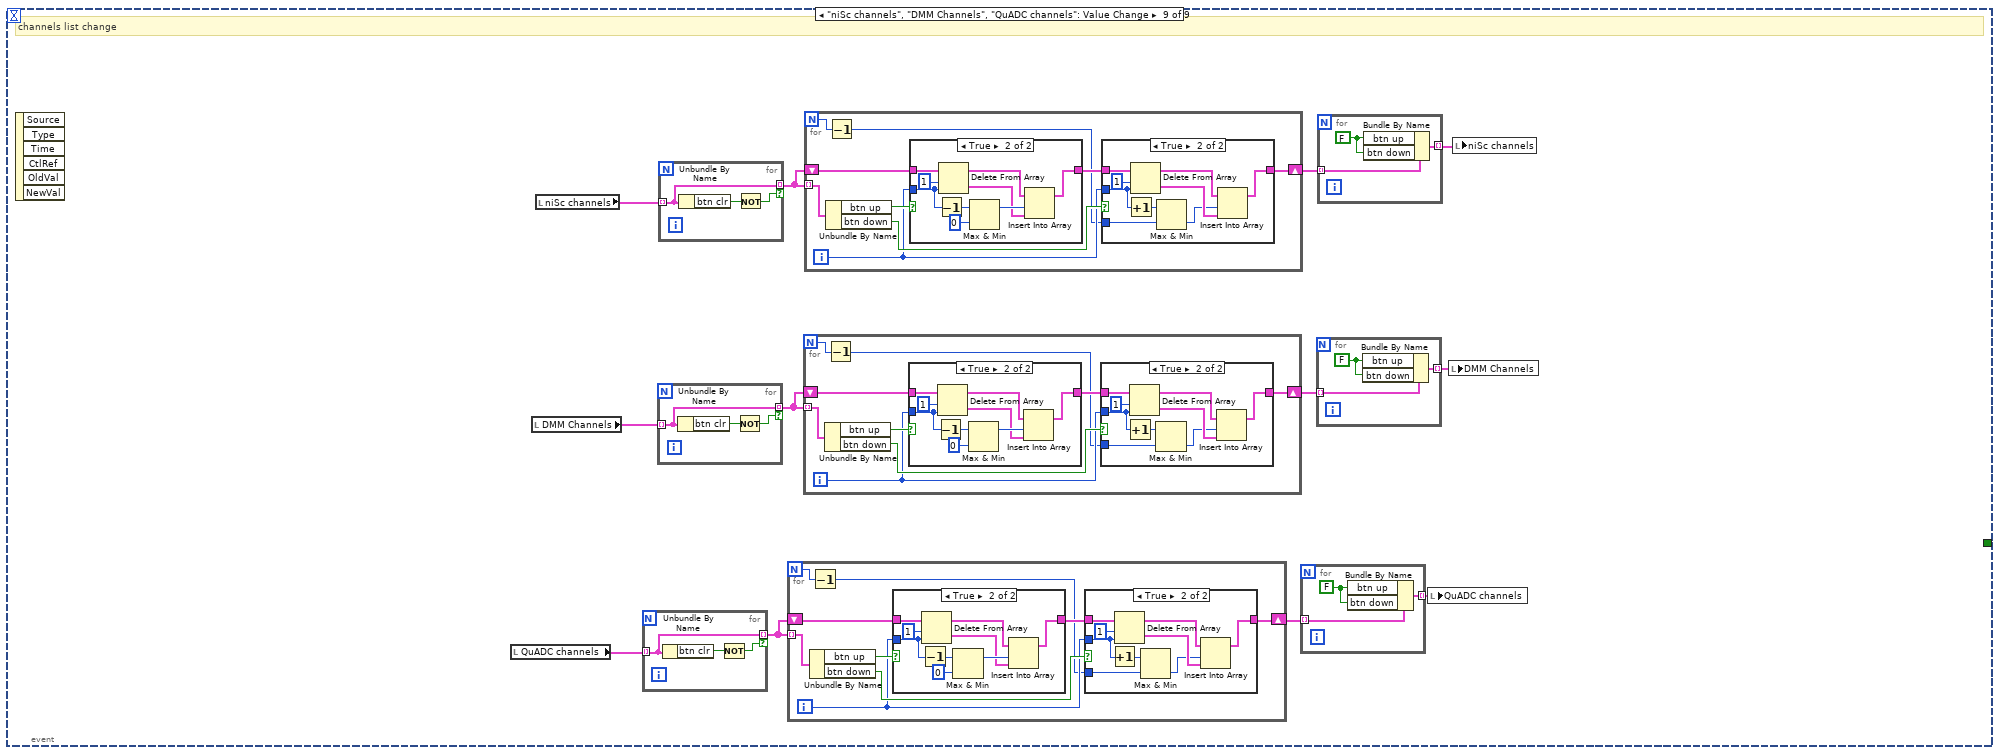
[diagram p14: hidden frame]
diagram:
  # "digitizer is busy"
  # "just for synchronisation"
  # "clear text string\nin this panel"
  # "register controls on this panel\nfor GUI control, but don't\ndiscard main panel ones (add to stack)"
  n1 = control-ref of="AWG VISA"() -> (w30:refnum<vi>)
  n2 = control-ref of="counter VISA"() -> (w27:refnum<vi>)
  n3 = control-ref of="btn selfcal"() -> (w32:refnum<vi>)
  n4 = control-ref of="AWG ext ref"() -> (w29:refnum<vi>)
  n5 = control-ref of="adcstr"() -> (w58:refnum<vi>)
  n6 = control-ref of="AWG type"() -> (w31:refnum<vi>)
  n7 = control-ref of="counter type"() -> (w28:refnum<vi>)
  n8 = Build Array(w58, w32, w31, w30, w29, w28, w27) -> (w57:refnum<vi>[])
  n9 = call "align_vi_panel.vi"() -> ("error out"=w26:errorcluster)  [unwired: 11 in]
  n10 = call "SGUI Register Controls.vi"("error in"=w26, "control references (empty)"=w57, "register mode (overwrite)"=SGUI_Assign_References_Mode."Add to stack") -> ("assigned ID"=w19:string, "error out"=w62:errorcluster)  [unwired: 14 in, 1 out]
  n11 = call-poly "SGUI Assign String With Tags.vi"("error in"=w62, "label(s) (empty)"="adcstr" ("string (empty)"), "string (empty)"="<bc=black><tc=cyan><al=left>" ("label(s) (empty)")) -> ("error out"=w56:errorcluster)  [unwired: 7 in, 1 out]
  n12 = control-ref of="btn selfcal"() -> (w50:refnum<vi>)
  n13 = control-ref of="btn test"() -> (w49:refnum<vi>)
  n14 = control-ref of="btn ok"() -> (w48:refnum<vi>)
  n15 = control-ref of="btn cancel"() -> (w47:refnum<vi>)
  n16 = Build Array(w50, w49, w48, w47) -> (w54:refnum<vi>[])
  n17 = Build Array(refnum<vi> refnum ("btn cancel")) -> (w52:refnum<vi>[])
  n18 = Bundle(w54) -> (w55:cluster{refnum<vi>[]})  [unwired: 1 in]
  n19 = Bundle(w52) -> (w53:cluster{refnum<vi>[]})  [unwired: 1 in]
  n20 = Build Array(w55, w53) -> (w51:cluster{refnum<vi>[]}[])
  n21 = call "SGUI Register Controls Groups.vi"("control groups"=w51, "error in"=w56, "groups names"="adcready\nadcbusy", "register mode (overwrite)"=SGUI_Assign_References_Mode."Add to stack") -> ("assigned ID"=w18:string, "error out"=w43:errorcluster)  [unwired: 14 in]
  n22 = call "SGUI Set Control Enabled State By Groups.vi"("error in"=w43, "group name to enable (none)"="adcready") -> ("error out"=w41:errorcluster)  [unwired: 8 in, 1 out]
  n23 = call <vilib>:"Clear Errors.vi"("error in (no error)"=w41) -> ("error out"=w14:errorcluster)  [unwired: 5 in, 1 out]
  n24 = Unbundle By Name("adc session in") -> ("QuADC session"=w2:T35, "exit mode"=w15:T1, "exit dly"=w16:dbl, "force rst?"=w17:bool, "type"=w40:T32, "niScope"=w79:T3, "3458A"=w75:T13, "dsdll"=w37:T28, "simadc"=w25:T33)
  n25 = call "ADC Reset Idle Timer.vi"("error in"=w14, "set busy (False)"=TRUE, "adc session in"="adc session in") -> ("error out"=w13:errorcluster, "adc session out"=w11:T2)  [unwired: 7 in]
  n26 = control-ref of="dsdll capt devs"() -> (w39:refnum<vi>)
  n27 = call "ADC Enumerate Devices.vi"("capture devices ring ref"=w39, "error in"=w13, "adc session in"=w11) -> ("error out"=w6:errorcluster, "adc session out"=→"adc session out":T2)  [unwired: 7 in]
  n28 = Unbundle By Name(w75) -> ("channels"=w74:T14[], "streaming mode"=w73:bool, "sync mode"=w72:T19, "sampling mode"=w71:T21, "idn mode"=w70:T20, "sync unit.VISA"=w69:refnum<visa-resource-name>, "sync unit.type"=w68:T16, "awg unit.type"=w67:T18, "awg unit.VISA"=w66:refnum<visa-resource-name>, "awg unit.enable 10MHz ref"=w65:bool, "measure temp.?"=w33:bool, "disable display?"=w20:bool, "aper mode"=w9:T27, "aper rules"=w7:dbl[][])
  n29 = Unbundle By Name(w2) -> ("channel cfg"=w1:T36[])
  n30 = Unbundle By Name(w79) -> ("channel cfg"=w78:T4[], "use streaming"=w77:bool, "ext. clock [Hz]"=w76:dbl)
  n31 = flat-sequence {
    tunnel: w40 -> [w80]
    tunnel: [w83] -> w4
    tunnel: [w82] -> w3
    frame #0 {
      n32 = To Long Integer(number=w80) -> (32bit integer=w81:i32)
      n33 = local write "Digitizer type"(w80) -> ()
      n34 = local write "tc cfg"(w81) -> ()
    }
    frame #1 {
      n35 = control-ref of="tc cfg"() -> (w82:refnum<vi>)
      n36 = control-ref of="Digitizer type"() -> (w83:refnum<vi>)
    }
  }
  n37 = Unbundle By Name(w25) -> ("channels"=w24:T34[], "range [V]"=w23:dbl, "Ts step [s]"=w22:dbl, "bit res"=w21:i32)
  n38 = local write "exit mode"(w15) -> ()
  n39 = local write "exit delay"(w16) -> ()
  n40 = local write "force rst"(w17) -> ()
  n41 = Unbundle By Name(w37) -> ("channels"=w36:i32, "device id"=w35:i32)
  n42 = local write "QuADC channels"(w1) -> ()
  n43 = call "ADC GUI Disable types.vi"("Tab ref"=w3, "Enum ref"=w4, "error in (no error)"=w6) -> ("error out"=w5:errorcluster)  [unwired: 8 in]
  n44 = while {
    tunnel: w5 -> [_]
    tunnel: [w84] -> w61
    stop <- w84 stop-if-true
    # "GUI Events Loop"
    n45 = event shown="[1] \"btn ok\", \"btn cancel\", \"btn test\", \"btn selfcal\": Value Change;  Panel Close" {
      selector: _ -> [_ _ _ _ _ _ _ _ _]
      dyn-events: _ -> [_ _ _ _ _ _ _ _ _]
      timeout: 333 -> [_ _ _ _ _ _ _ _ _]
      tunnel: [_ w137 _ _ _ _ _ _ _] -> w84
      event Timeout {
        # "enable/disable DMM aux HW setup"
        # "HW has selfcal option?"
        # "select ADC config tab"
        # "show mode description"
        n46 = event-data() -> ()  [unwired: 1 in, 3 out]
        n47 = local read "dmm sync mode"() -> (w103:T19)
        n48 = local read "Digitizer type"() -> (w101:T32)
        n49 = Bundle By Name(cluster=T13 {"channels"=[], "sync unit"={"VISA"="", "type"=enum."Picotest U6200A"}, "awg unit"={"type"=enum."Agilent 331xxA to 332xxA", "VISA"="", "enable 10MHz ref"=FALSE}, "sync mode"=enum."MASTER-SLAVE, MASTER clocked by TIMER", "streaming mode"=FALSE, "idn mode"=enum."Auto", "sampling mode"=enum."DCV", "Ts [s]"=0.0, "sample memory [B]"=0, "proc setup"={"channel id"=0, "packet size [smpl]"=0, "current timeout [s]"=0.0, "blk2blk timeout [s]"=0.0, "event time"=timestamp(0 s since 1904-01-01), "stop notifier"=refnum, "data queues"=[], "proc refs"=[], "bus semaphore"=refnum}, "sample size [B]"=0, "sample count"=0, "aux data"={"channel id"=0, "valid?"=[], "gain [V]"=[], "timestamp [s]"=[], "Ts [s]"=0.0, "abs timestamp"=timestamp(0 s since 1904-01-01), "t [deg C]"=[]}, "ranges [V]"=[], "aperture [s]"=0.0, "LEVEL trigger"={"edge"=enum."POS", "level [V]"=0.0, "coupling"=enum."DC"}, "trigger mode"=enum."AUTO", "measure temp.?"=FALSE, "disp mesages"=[], "shared bus?"=FALSE, "disable display?"=FALSE, "aper mode"=enum."Manual", "aper rules"=[]} ("digitizer session"), "sync mode"=w103) -> (w92:T13)
        n50 = To Long Integer(number=w101) -> (32bit integer=w100:i32)
        n51 = local read "adc session out"() -> (w99:T2)
        n52 = local write "tc cfg"(w100) -> ()
        n53 = Bundle By Name(cluster=w99, "type"=w101, "3458A"=w92) -> (w98:T2)
        n54 = call "3458A Check Needed Aux HW.vi"("digitizer session"=w92) -> ("uses AWG clocking?"=w91:bool, "uses counter?"=w88:bool)  [unwired: 13 in, 4 out]
        n55 = call "ADC Get Capabilities.vi"("adc session in"=w98) -> ("error out"=w93:errorcluster, "capabilities"=w97:T45)  [unwired: 8 in, 1 out]
        n56 = call "ADC GUI Get Info.vi"("adc session"=w98) -> ("configuration description"=w102:string)
        n57 = call "SGUI Set Control Enabled State By Label.vi"("labels (empty)"="AWG type\nAWG ext ref\nAWG VISA", "Enabled? (False)"=w91) -> ("error out"=w89:errorcluster)  [unwired: 8 in, 1 out]
        n58 = Unbundle By Name(w97) -> ("has selfcal?"=w96:bool)
        n59 = local write "Description"(w102) -> ()
        n60 = call "SGUI Set Control Enabled State By Label.vi"("error in"=w93, "labels (empty)"="btn selfcal", "Enabled? (False)"=w96) -> ("error out"=w94:errorcluster)  [unwired: 7 in, 1 out]
        n61 = call "SGUI Set Control Enabled State By Label.vi"("error in"=w89, "labels (empty)"="counter type\ncounter VISA", "Enabled? (False)"=w88) -> ("error out"=w86:errorcluster)  [unwired: 7 in, 1 out]
        n62 = call <vilib>:"Clear Errors.vi"("error in (no error)"=w94) -> ()  [unwired: 5 in, 2 out]
        n63 = call <vilib>:"Clear Errors.vi"("error in (no error)"=w86) -> ()  [unwired: 5 in, 2 out]
      }
      event "btn ok", "btn cancel", "btn test", "btn selfcal": Value Change; Panel Close {
        # "OK - update setup"
        # "OK or Cancel or Exit"
        n64 = event-data() -> ()  [unwired: 1 in, 3 out]
        n65 = local read "dmm aper rules"() -> (w111:string[][])
        n66 = for {
          tunnel: w111 -> [w157] mode=indexing
          tunnel: [w156] -> w110 mode=indexing
          n67 = for {
            tunnel: w157 -> [w160] mode=indexing
            tunnel: [w159] -> w156 mode=indexing
            n68 = Scan Value(string=w160, format string="%p") -> (value=w159:dbl)  [unwired: 1 in, 1 out]
          }
        }
        n69 = local read "DMM Channels"() -> (w152:T14[])
        n70 = local read "dmm stream"() -> (w151:bool)
        n71 = local read "dmm sync mode"() -> (w150:T19)
        n72 = local read "dmm smpl mode"() -> (w149:T21)
        n73 = local read "dmm idn mode"() -> (w148:T20)
        n74 = local read "counter VISA"() -> (w147:refnum<visa-resource-name>)
        n75 = local read "counter type"() -> (w146:T16)
        n76 = local read "AWG type"() -> (w145:T18)
        n77 = local read "AWG VISA"() -> (w144:refnum<visa-resource-name>)
        n78 = local read "AWG ext ref"() -> (w143:bool)
        n79 = local read "dmm meas t"() -> (w126:bool)
        n80 = local read "dmm disable disp"() -> (w116:bool)
        n81 = local read "dmm aper mode"() -> (w112:T27)
        n82 = local read "adc session out"() -> (w132:T2)
        n83 = local read "Sampling period step [s]"() -> (w120:dbl)
        n84 = local read "dsdll capt devs"() -> (w134:u16)
        n85 = local read "dsdll channels"() -> (w133:i32)
        n86 = local read "simadc chn cfg"() -> (w122:T34[])
        n87 = local read "simadc bitres"() -> (w117:i32)
        n88 = local read "niSc channels"() -> (w155:T4[])
        n89 = local read "niSc streaming"() -> (w154:bool)
        n90 = local read "niSc ext clock"() -> (w153:dbl)
        n91 = Unbundle By Name(w132) -> ("dsdll"=w131:T28, "3458A"=w130:T13, "niScope"=w129:T3, "simadc"=w123:T33, "QuADC session"=w109:T35)
        n92 = local read "Range [V]"() -> (w121:dbl)
        n93 = Bundle By Name(cluster=w130, "channels"=w152, "streaming mode"=w151, "sync mode"=w150, "sampling mode"=w149, "idn mode"=w148, "sync unit.VISA"=w147, "sync unit.type"=w146, "awg unit.type"=w145, "awg unit.VISA"=w144, "awg unit.enable 10MHz ref"=w143, "measure temp.?"=w126, "disable display?"=w116, "aper mode"=w112, "aper rules"=w110) -> (w141:T13)
        n94 = Bundle By Name(cluster=w131, "device id"=w134, "channels"=w133) -> (w135:T28)
        n95 = Bundle By Name(cluster=w123, "channels"=w122, "range [V]"=w121, "Ts step [s]"=w120, "time [s]"=0.0, "bit res"=w117) -> (w118:T33)
        n96 = Bundle By Name(cluster=w129, "channels"=0, "channel cfg"=w155, "use streaming"=w154, "ext. clock [Hz]"=w153) -> (w142:T3)
        n97 = local read "Digitizer type"() -> (w140:T32)
        n98 = local read "exit mode"() -> (w113:T1)
        n99 = local read "exit delay"() -> (w114:dbl)
        n100 = local read "QuADC channels"() -> (w107:T36[])
        n101 = local read "force rst"() -> (w115:bool)
        n102 = Bundle By Name(cluster=w109, "channels"=0, "channel cfg"=w107, "use streaming"=TRUE) -> (w105:T35)
        n103 = Bundle By Name(cluster=w132, "exit mode"=w113, "exit dly"=w114, "force rst?"=w115, "modified?"=TRUE, "type"=w140, "niScope"=w142, "3458A"=w141, "dsdll"=w135, "simadc"=w118, "QuADC session"=w105) -> (w127:T2)
        n104 = Select(t=w127, s="btn ok", f=w132) -> (s? t:f=w138:T2)
        n105 = local write "adc session out"(w138) -> ()
        n106 = case shown="True" "btn selfcal" {
          tunnel: w127 -> [_ w167]
          frame False {
          }
          frame True {
            # "controls to ready"
            # "controls to busy"
            # "clear idn string"
            # "SELFCAL"
            n107 = invoke on="error out" class="Clust (strict)" method="Reinit To Default"() -> (error out=w168:errorcluster)  [unwired: 3 in, 2 out]
            n108 = call-poly "SGUI Assign String With Tags.vi"("error in"=w168, "label(s) (empty)"="adcstr", "string (empty)"="") -> ("error out"=w171:errorcluster)  [unwired: 7 in, 1 out]
            n109 = call "SGUI Set Control Enabled State By Groups.vi"("error in"=w171, "group name to enable (none)"="adcbusy") -> ("error out"=w172:errorcluster)  [unwired: 8 in, 1 out]
            n110 = call "ADC Initialize Virtual Channels.vi"("error in"=w172, "Reset? (False)"=TRUE, "adc session in"=w167) -> ("error out"=w177:errorcluster, "adc session out"=w165:T2, "all instruments idn strings"=w161:string[])  [unwired: 4 in, 2 out]
            n111 = for {
              tunnel: w161 -> [w186] mode=indexing
              tunnel: [w184] -> w179 mode=indexing
              n112 = Concatenate Strings("<b>" ("string"), w186, "\r") -> (w184:string)
            }
            n113 = Concatenate Strings(w179) -> (w180:string)
            n114 = call <vilib>:"Trim Whitespace.vi"("string"=w180) -> ("trimmed string"=w181:string)  [unwired: 1 in]
            n115 = call-poly "SGUI Assign String With Tags.vi"("error in"=w177, "label(s) (empty)"="adcstr", "string (empty)"=w181) -> ("error out"=w166:errorcluster)  [unwired: 7 in, 1 out]
            n116 = call "ADC Selfcal Virtual Channels.vi"("error in"=w166, "adc session in"=w165) -> ("error out"=w163:errorcluster, "adc session out"=w164:T2)  [unwired: 8 in]
            n117 = call "ADC Close Virtual Channels.vi"("error in"=w163, "adc session in"=w164) -> ("error out"=w174:errorcluster, "adc session out"=w162:T2)  [unwired: 8 in]
            n118 = call "SGUI Set Control Enabled State By Groups.vi"("error in"=w174, "group name to enable (none)"="adcready") -> ("error out"=w175:errorcluster)  [unwired: 8 in, 1 out]
            n119 = local write "adc session out"(w162) -> ()
            n120 = local write "error out"(w175) -> ()
          }
        }
        n121 = case shown="True" "btn test" {
          tunnel: w127 -> [_ w215]
          frame False {
          }
          frame True {
            # "controls to ready"
            # "controls to busy"
            # "clear idn string"
            # "IDENTIFY and TEST instruments"
            n122 = invoke on="error out" class="Clust (strict)" method="Reinit To Default"() -> (error out=w214:errorcluster)  [unwired: 3 in, 2 out]
            n123 = call-poly "SGUI Assign String With Tags.vi"("error in"=w214, "label(s) (empty)"="adcstr", "string (empty)"="") -> ("error out"=w211:errorcluster)  [unwired: 7 in, 1 out]
            n124 = call "SGUI Set Control Enabled State By Groups.vi"("error in"=w211, "group name to enable (none)"="adcbusy") -> ("error out"=w195:errorcluster)  [unwired: 8 in, 1 out]
            n125 = call "dialog_wait.vi"("error in"=w195, "message string"="Please wait, initalizing digitizers ...") -> ("error out"=w194:errorcluster, "reference out"=w191:refnum<vi>)  [unwired: 8 in]
            n126 = call "ADC Initialize Virtual Channels.vi"("error in"=w194, "Reset? (False)"=TRUE, "adc session in"=w215) -> ("error out"=w199:errorcluster, "adc session out"=w189:T2, "all instruments idn strings"=w187:string[])  [unwired: 4 in, 2 out]
            n127 = for {
              tunnel: w187 -> [w223] mode=indexing
              tunnel: [w221] -> w206 mode=indexing
              n128 = Concatenate Strings("<b><tc=cyan>" ("string"), w223, "\r") -> (w221:string)
            }
            n129 = Unbundle By Name(w199) -> ("source"=w201:string)
            n130 = Concatenate Strings("<b><tc=red>" ("string"), w201) -> (w198:string)
            n131 = Concatenate Strings(w206) -> (w205:string)
            n132 = call <vilib>:"Trim Whitespace.vi"("string"=w205) -> ("trimmed string"=w197:string)  [unwired: 1 in]
            n133 = Unbundle By Name(w189) -> ("exit mode"=w188:T1)
            n134 = Select(t=w198, s=w199, f=w197) -> (s? t:f=w196:string)
            n135 = call-poly "SGUI Assign String With Tags.vi"("error in"=w199, "label(s) (empty)"="adcstr", "string (empty)"=w196) -> ("error out"=w203:errorcluster)  [unwired: 7 in, 1 out]
            n136 = case shown="\"Immediate reset\"" w188 {
              tunnel: w203 -> [w216 w218]
              tunnel: [w216 w217] -> w202
              frame Default {
              }
              frame "Immediate reset" {
                n137 = call "Wait (ms) With Conditional Error Input.vi"("error in (no error)"=w218, "milliseconds to wait"=u32 1000) -> ("error out"=w217:errorcluster)  [unwired: 8 in, 1 out]
              }
            }
            n138 = call "ADC Close Virtual Channels.vi"("error in"=w202, "adc session in"=w189) -> ("error out"=w192:errorcluster, "adc session out"=w190:T2)  [unwired: 8 in]
            n139 = call "SGUI Set Control Enabled State By Groups.vi"("error in"=w192, "group name to enable (none)"="adcready") -> ("error out"=w209:errorcluster)  [unwired: 8 in, 1 out]
            n140 = call "dialog_wait_close.vi"("error in"=w192, "async vi ref"=w191) -> ()  [unwired: 2 in]
            n141 = local write "adc session out"(w190) -> ()
            n142 = local write "error out"(w209) -> ()
          }
        }
        n143 = Compound Arithmetic op=OR("btn selfcal", "btn test") -> (invert w137:bool)
      }
      event "tc cfg": Value Change {
        # "Change HW selection by tabs"
        n144 = event-data() -> ("NewVal"=w225:T43)  [unwired: 1 in, 5 out]
        n145 = To Unsigned Word Integer(number=w225) -> (unsigned 16bit integer=w224:u16)
        n146 = property on="Digitizer type" class="Enum (strict)"("Val(Sgnl)"=w224) -> ()  [unwired: 2 in, 2 out]
      }
      event "btn clr dmm", "btn clr niScope": Value Change {
        # "clear channels lists"
        n147 = event-data() -> ()  [unwired: 1 in, 6 out]
        n148 = case shown="False" "btn clr niScope" {
          frame False {
            # "clear 3458A chn list"
            n149 = invoke on="DMM Channels" class="Arr" method="Reinit To Default"() -> ()  [unwired: 3 in, 3 out]
          }
          frame True {
            # "clear niScope chn list"
            n150 = invoke on="niSc channels" class="Arr" method="Reinit To Default"() -> ()  [unwired: 3 in, 3 out]
          }
        }
      }
      event "btn rem last dmm", "btn rem last niScope": Value Change {
        # "Remove last item from channel list"
        n151 = event-data() -> ()  [unwired: 1 in, 6 out]
        n152 = case shown="False" "btn rem last dmm" {
          frame False {
            n153 = local read "niSc channels"() -> (w231:T4[])
            n154 = Array Size(array=w231) -> (size(s)=w230:i32)
            n155 = Decrement(x=w230) -> (x-1=w229:i32)
            n156 = Array Subset(array=w231, length=w229) -> (w228:T4[])  [unwired: 1 in]
            n157 = local write "niSc channels"(w228) -> ()
          }
          frame True {
            n158 = local read "DMM Channels"() -> (w235:T14[])
            n159 = Array Size(array=w235) -> (size(s)=w234:i32)
            n160 = Decrement(x=w234) -> (x-1=w233:i32)
            n161 = Array Subset(array=w235, length=w233) -> (w232:T14[])  [unwired: 1 in]
            n162 = local write "DMM Channels"(w232) -> ()
          }
        }
      }
      event "btn dsdll enum": Value Change {
        # "Update DSDLL device list"
        n163 = event-data() -> ()  [unwired: 1 in, 6 out]
        n164 = local read "Digitizer type"() -> (w236:T32)
        n165 = local read "adc session out"() -> (w238:T2)
        n166 = Bundle By Name(cluster=w238, "type"=w236) -> (w239:T2)
        n167 = control-ref of="dsdll capt devs"() -> (w240:refnum<vi>)
        n168 = call "ADC Enumerate Devices.vi"("capture devices ring ref"=w240, "adc session in"=w239) -> ("error out"=w237:errorcluster)  [unwired: 8 in, 1 out]
        n169 = call <vilib>:"Clear Errors.vi"("error in (no error)"=w237) -> ()  [unwired: 5 in, 2 out]
      }
      event "btn sim clr": Value Change {
        # "clear simulated ADC list"
        n170 = event-data() -> ()  [unwired: 1 in, 6 out]
        n171 = invoke on="simadc chn cfg" class="Arr" method="Reinit To Default"() -> ()  [unwired: 3 in, 3 out]
      }
      event "simadc chn cfg": Value Change {
        # "value changed in the sim ADC setup"
        n172 = event-data() -> ()  [unwired: 1 in, 6 out]
        n173 = local read "simadc chn cfg"() -> (w245:T34[])
        n174 = Bundle By Name(cluster=T33 {"channels"=[], "range [V]"=0.0, "Ts step [s]"=0.0, "time [s]"=0.0, "fs [Hz]"=0.0, "count"=0, "smpl offset"=0, "set count"=0, "bit res"=0} ("Cluster"), "channels"=w245) -> (w244:T33)
        n175 = call "SimAdc Clear Channels.ctl"("simadc in"=w244) -> ("error out"=w243:errorcluster, "simadc out"=w242:T33)  [unwired: 9 in]
        n176 = Unbundle By Name(w242) -> ("channels"=w241:T34[])
        n177 = call <vilib>:"Clear Errors.vi"("error in (no error)"=w243) -> ()  [unwired: 5 in, 2 out]
        n178 = local write "simadc chn cfg"(w241) -> ()
      }
      event "niSc channels", "DMM Channels", "QuADC channels": Value Change {
        # "channels list change"
        n179 = event-data() -> ()  [unwired: 1 in, 6 out]
        n180 = local read "QuADC channels"() -> (w250:T36[])
        n181 = local read "DMM Channels"() -> (w251:T14[])
        n182 = local read "niSc channels"() -> (w258:T4[])
        n183 = for {
          tunnel: w250 -> [w293] mode=indexing
          tunnel: [w293] -> w249 mode=indexing if=w291
          n184 = Unbundle By Name(w293) -> ("btn clr"=w292:bool)
          n185 = Not(x=w292) -> (.not. x?=w291:bool)
        }
        n186 = for {
          tunnel: w251 -> [w328] mode=indexing
          tunnel: [w328] -> w252 mode=indexing if=w326
          n187 = Unbundle By Name(w328) -> ("btn clr"=w327:bool)
          n188 = Not(x=w327) -> (.not. x?=w326:bool)
        }
        n189 = for {
          tunnel: w258 -> [w363] mode=indexing
          tunnel: [w363] -> w257 mode=indexing if=w361
          n190 = Unbundle By Name(w363) -> ("btn clr"=w362:bool)
          n191 = Not(x=w362) -> (.not. x?=w361:bool)
        }
        n192 = for {
          N -> [w264]
          tunnel: w249 -> [w269] mode=indexing
          shift-right: [w262] -> w248
          shift-left: w249 -> [w268]
          i -> [w265]
          n193 = Unbundle By Name(w269) -> ("btn up"=w270:bool, "btn down"=w266:bool)
          n194 = Decrement(x=w264) -> (x-1=w263:i32)
          n195 = case shown="True" w270 {
            tunnel: w268 -> [w281 w290]
            tunnel: w265 -> [_ w288]
            tunnel: [w281 w283] -> w267
            frame False {
            }
            frame True {
              n196 = Decrement(x=w288) -> (x-1=w282:i32)
              n197 = Delete From Array(array=w290, length=1, index=w288) -> (deleted portion=w284:T36[], array with subset deleted=w285:T36[])
              n198 = Max & Min(x=w282, y=0) -> (max(x,y)=w286:i32)  [unwired: 1 out]
              n199 = Insert Into Array(array=w285, index=w286, new element=w284) -> (w283:T36[])
            }
          }
          n200 = case shown="True" w266 {
            tunnel: w267 -> [w271 w280]
            tunnel: w265 -> [_ w278]
            tunnel: [w271 w275] -> w262
            tunnel: w263 -> [_ w274]
            frame False {
            }
            frame True {
              n201 = Increment(x=w278) -> (x+1=w272:i32)
              n202 = Delete From Array(array=w280, length=1, index=w278) -> (deleted portion=w276:T36[], array with subset deleted=w277:T36[])
              n203 = Max & Min(x=w272, y=w274) -> (min(x,y)=w273:i32)  [unwired: 1 out]
              n204 = Insert Into Array(array=w277, index=w273, new element=w276) -> (w275:T36[])
            }
          }
        }
        n205 = for {
          N -> [w299]
          tunnel: w252 -> [w304] mode=indexing
          shift-right: [w297] -> w253
          shift-left: w252 -> [w303]
          i -> [w300]
          n206 = Unbundle By Name(w304) -> ("btn up"=w305:bool, "btn down"=w301:bool)
          n207 = Decrement(x=w299) -> (x-1=w298:i32)
          n208 = case shown="True" w305 {
            tunnel: w303 -> [w316 w325]
            tunnel: w300 -> [_ w323]
            tunnel: [w316 w318] -> w302
            frame False {
            }
            frame True {
              n209 = Decrement(x=w323) -> (x-1=w317:i32)
              n210 = Delete From Array(array=w325, length=1, index=w323) -> (deleted portion=w319:T14[], array with subset deleted=w320:T14[])
              n211 = Max & Min(x=w317, y=0) -> (max(x,y)=w321:i32)  [unwired: 1 out]
              n212 = Insert Into Array(array=w320, index=w321, new element=w319) -> (w318:T14[])
            }
          }
          n213 = case shown="True" w301 {
            tunnel: w302 -> [w306 w315]
            tunnel: w300 -> [_ w313]
            tunnel: [w306 w310] -> w297
            tunnel: w298 -> [_ w309]
            frame False {
            }
            frame True {
              n214 = Increment(x=w313) -> (x+1=w307:i32)
              n215 = Delete From Array(array=w315, length=1, index=w313) -> (deleted portion=w311:T14[], array with subset deleted=w312:T14[])
              n216 = Max & Min(x=w307, y=w309) -> (min(x,y)=w308:i32)  [unwired: 1 out]
              n217 = Insert Into Array(array=w312, index=w308, new element=w311) -> (w310:T14[])
            }
          }
        }
        n218 = for {
          N -> [w334]
          tunnel: w257 -> [w339] mode=indexing
          shift-right: [w332] -> w256
          shift-left: w257 -> [w338]
          i -> [w335]
          n219 = Unbundle By Name(w339) -> ("btn up"=w340:bool, "btn down"=w336:bool)
          n220 = Decrement(x=w334) -> (x-1=w333:i32)
          n221 = case shown="True" w340 {
            tunnel: w338 -> [w351 w360]
            tunnel: w335 -> [_ w358]
            tunnel: [w351 w353] -> w337
            frame False {
            }
            frame True {
              n222 = Decrement(x=w358) -> (x-1=w352:i32)
              n223 = Delete From Array(array=w360, length=1, index=w358) -> (deleted portion=w354:T4[], array with subset deleted=w355:T4[])
              n224 = Max & Min(x=w352, y=0) -> (max(x,y)=w356:i32)  [unwired: 1 out]
              n225 = Insert Into Array(array=w355, index=w356, new element=w354) -> (w353:T4[])
            }
          }
          n226 = case shown="True" w336 {
            tunnel: w337 -> [w341 w350]
            tunnel: w335 -> [_ w348]
            tunnel: [w341 w345] -> w332
            tunnel: w333 -> [_ w344]
            frame False {
            }
            frame True {
              n227 = Increment(x=w348) -> (x+1=w342:i32)
              n228 = Delete From Array(array=w350, length=1, index=w348) -> (deleted portion=w346:T4[], array with subset deleted=w347:T4[])
              n229 = Max & Min(x=w342, y=w344) -> (min(x,y)=w343:i32)  [unwired: 1 out]
              n230 = Insert Into Array(array=w347, index=w343, new element=w346) -> (w345:T4[])
            }
          }
        }
        n231 = for {
          tunnel: w248 -> [w261] mode=indexing
          tunnel: [w259] -> w247 mode=indexing
          w260 = FALSE ("btn up")
          n232 = Bundle By Name(cluster=w261, "btn up"=w260, "btn down"=w260) -> (w259:T36)
        }
        n233 = for {
          tunnel: w253 -> [w296] mode=indexing
          tunnel: [w294] -> w254 mode=indexing
          w295 = FALSE ("btn up")
          n234 = Bundle By Name(cluster=w296, "btn up"=w295, "btn down"=w295) -> (w294:T14)
        }
        n235 = for {
          tunnel: w256 -> [w331] mode=indexing
          tunnel: [w329] -> w255 mode=indexing
          w330 = FALSE ("btn up")
          n236 = Bundle By Name(cluster=w331, "btn up"=w330, "btn down"=w330) -> (w329:T4)
        }
        n237 = local write "QuADC channels"(w247) -> ()
        n238 = local write "DMM Channels"(w254) -> ()
        n239 = local write "niSc channels"(w255) -> ()
      }
    }
  }
  n240 = local write "niSc channels"(w78) -> ()
  n241 = local write "niSc streaming"(w77) -> ()
  n242 = local write "niSc ext clock"(w76) -> ()
  n243 = local write "simadc chn cfg"(w24) -> ()
  n244 = local write "Range [V]"(w23) -> ()
  n245 = local write "Sampling period step [s]"(w22) -> ()
  n246 = local write "simadc bitres"(w21) -> ()
  n247 = local write "DMM Channels"(w74) -> ()
  n248 = local write "dmm stream"(w73) -> ()
  n249 = local write "dmm sync mode"(w72) -> ()
  n250 = local write "dmm smpl mode"(w71) -> ()
  n251 = local write "dmm idn mode"(w70) -> ()
  n252 = local write "counter VISA"(w69) -> ()
  n253 = local write "counter type"(w68) -> ()
  n254 = local write "AWG type"(w67) -> ()
  n255 = local write "AWG VISA"(w66) -> ()
  n256 = local write "AWG ext ref"(w65) -> ()
  n257 = local write "dmm meas t"(w33) -> ()
  n258 = local write "dmm disable disp"(w20) -> ()
  n259 = local write "dmm aper mode"(w9) -> ()
  n260 = local write "dsdll channels"(w36) -> ()
  n261 = local write "dsdll capt devs"(w35) -> ()
  n262 = for {
    tunnel: [w365] -> w8 mode=indexing
    tunnel: w7 -> [w364] mode=indexing
    n263 = for {
      tunnel: [w367] -> w365 mode=indexing
      tunnel: w364 -> [w366] mode=indexing
      n264 = Format Into String(format string="%#_4p" ("delimiter (Tab)"), w366) -> (resulting string=w367:string)  [unwired: 2 in, 1 out]
    }
  }
  n265 = local write "dmm aper rules"(w8) -> ()
  n266 = flat-sequence {
    tunnel: w61 -> [_]
    tunnel: w19 -> [w374]
    tunnel: w18 -> [w373]
    frame #0 {
      w375 = SGUI_Assign_References_Mode."Release ID" ("register mode (overwrite)")
      # "unregister controls\nof this panel"
      # "unregister controls of this panel"
      # "on panel close action"
      n267 = local read "adc session out"() -> (w371:T2)
      n268 = call "ADC Reset Idle Timer.vi"("set busy (False)"=FALSE, "adc session in"=w371) -> ("error out"=w372:errorcluster, "adc session out"=w370:T2)  [unwired: 8 in]
      n269 = local write "adc session out"(w370) -> ()
      n270 = call "SGUI Register Controls.vi"("error in"=w372, "register mode (overwrite)"=w375, "controls ID (empty)"=w374) -> ("error out"=w377:errorcluster)  [unwired: 14 in, 2 out]
      n271 = call "SGUI Register Controls Groups.vi"("error in"=w377, "register mode (overwrite)"=w375, "controls ID (empty)"=w373) -> ("error out"=w376:errorcluster)  [unwired: 15 in, 1 out]
      n272 = call <vilib>:"Clear Errors.vi"("error in (no error)"=w376) -> ()  [unwired: 5 in, 2 out]
    }
  }
  "error out" <- "error in"
  "adcstr" <- "" ("adcstr")
